vi "Distribution Example 2014yr.vi"() -> ()   [LabVIEW 2014]
uses:
  <vilib>/addons/database/Connection.llb/DB Tools Open Connec (Path).vi
  <userlib>/_OpenG.lib/array/array.llb/Search 1D Array (I32)__ogtk.vi
  <userlib>/_OpenG.lib/array/array.llb/Search 1D Array (Boolean)__ogtk.vi
  <vilib>/addons/database/NI_Database_API.lvlib
panel:
  out "size(s)":i32
  out "sum":i32
  out "Annual Distribution":cluster{dbl[], dbl[]}[](graph)
  out "Table 2":string[][](table)=[["34", "74", "23", "35", "23", "26", "74", "74", "21", "39", "61", "83"], ["73", "24", "75", "87", "42", "34", "35", "76", "52", "43", "43", "3"], ["36", "25", "12", "34", "24", "74", "73", "54", "88", "64", "90", "62"]]
  out "output array":i32[](array[numeric])
  out "Array 2":i32[](array[numeric])
  out "Array":i32[](array[numeric])
  out "data":string[][](table)
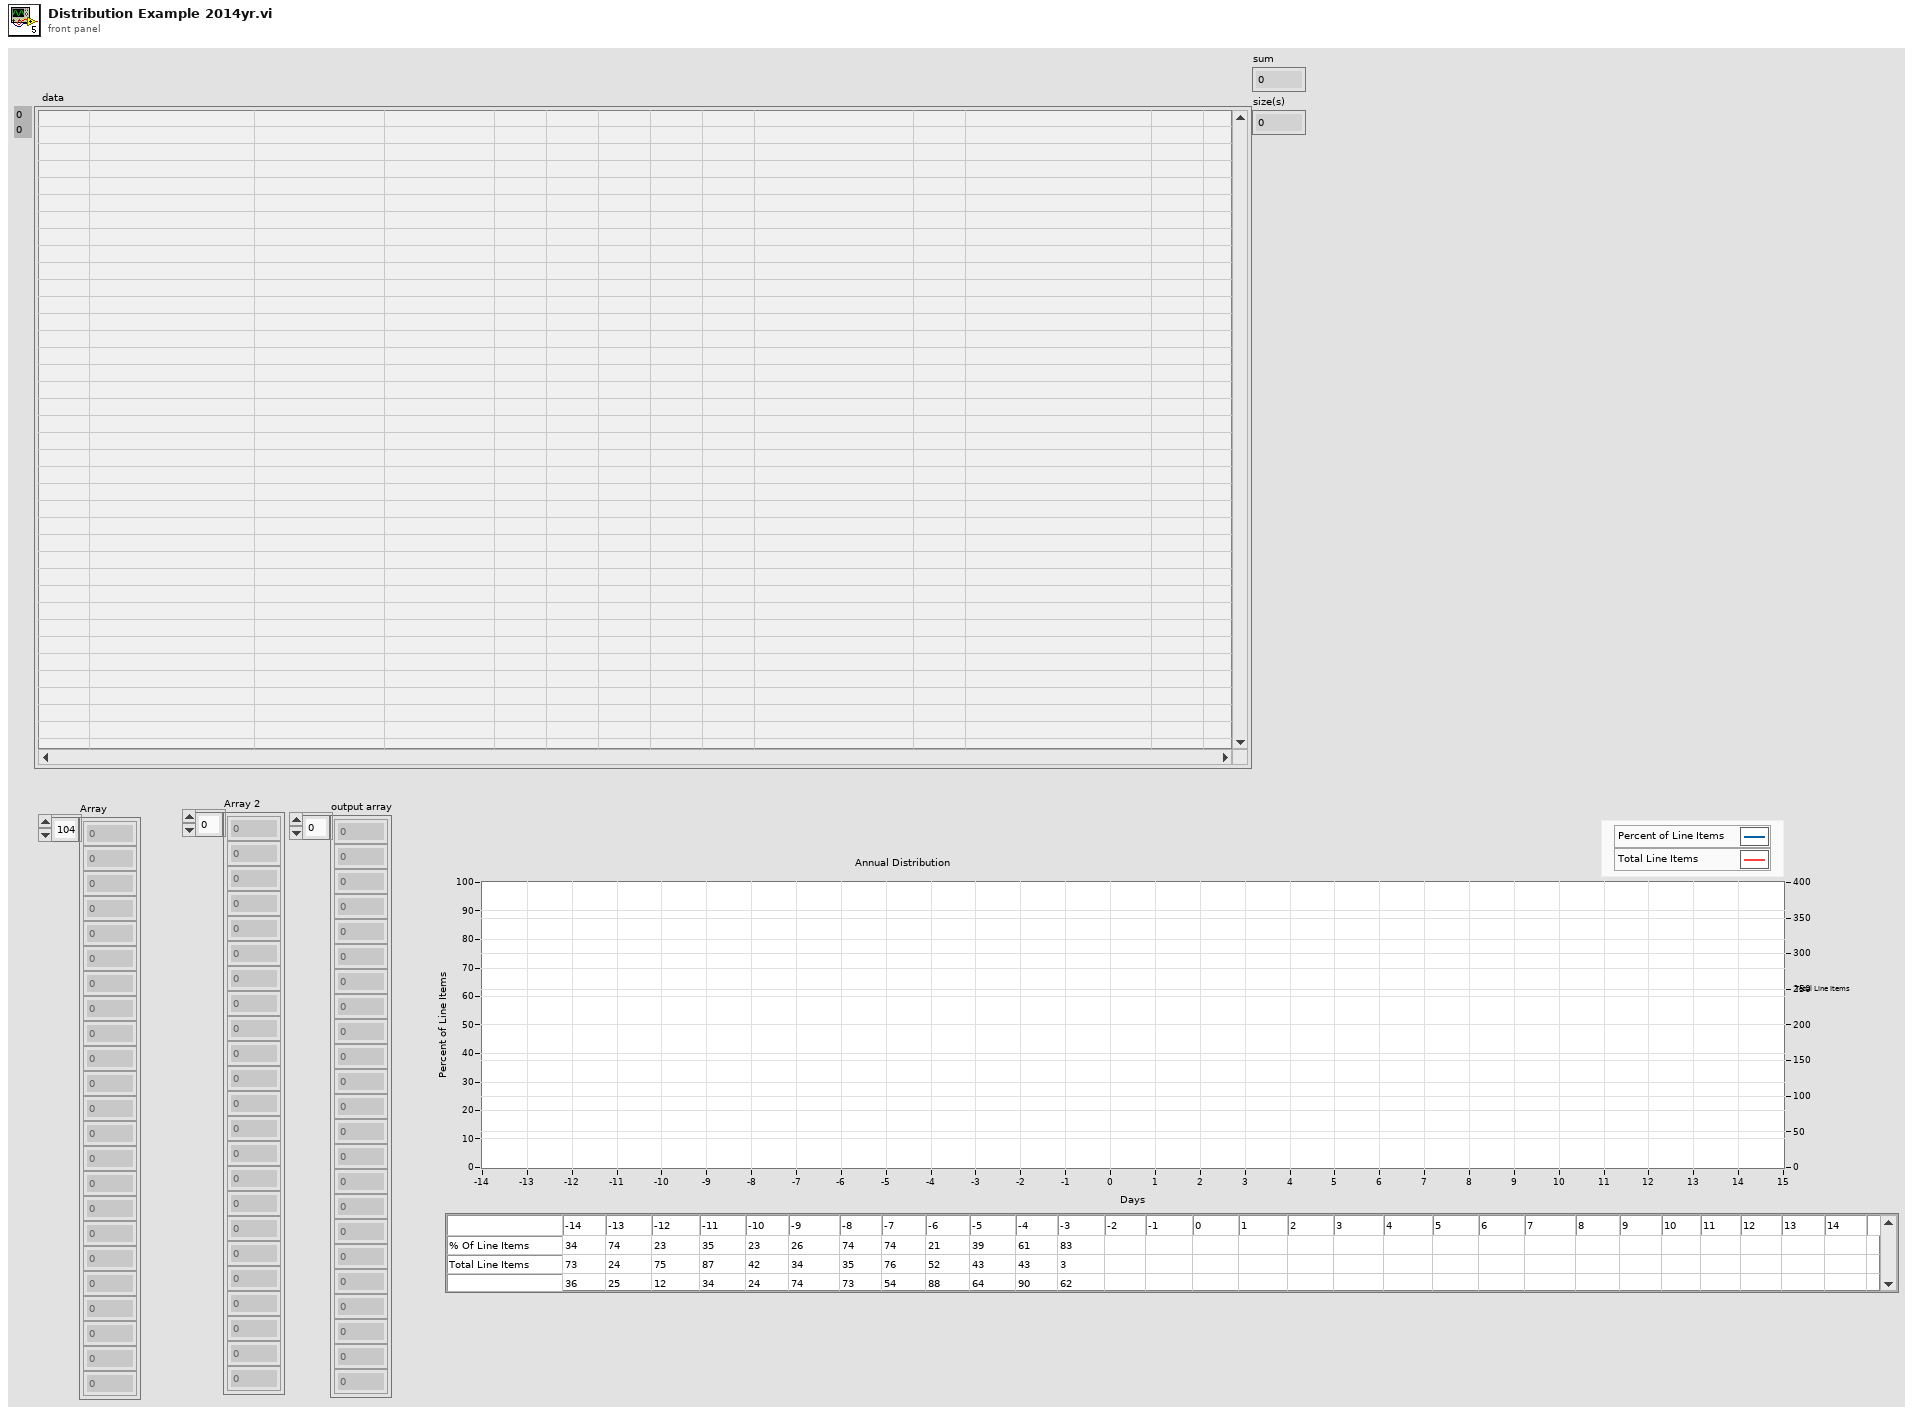
[diagram p1: front panel]
types:
  T1 = typedef "NI_Database_API.lvlib/Conn ObjectReference.ctl" = refnum<k1>
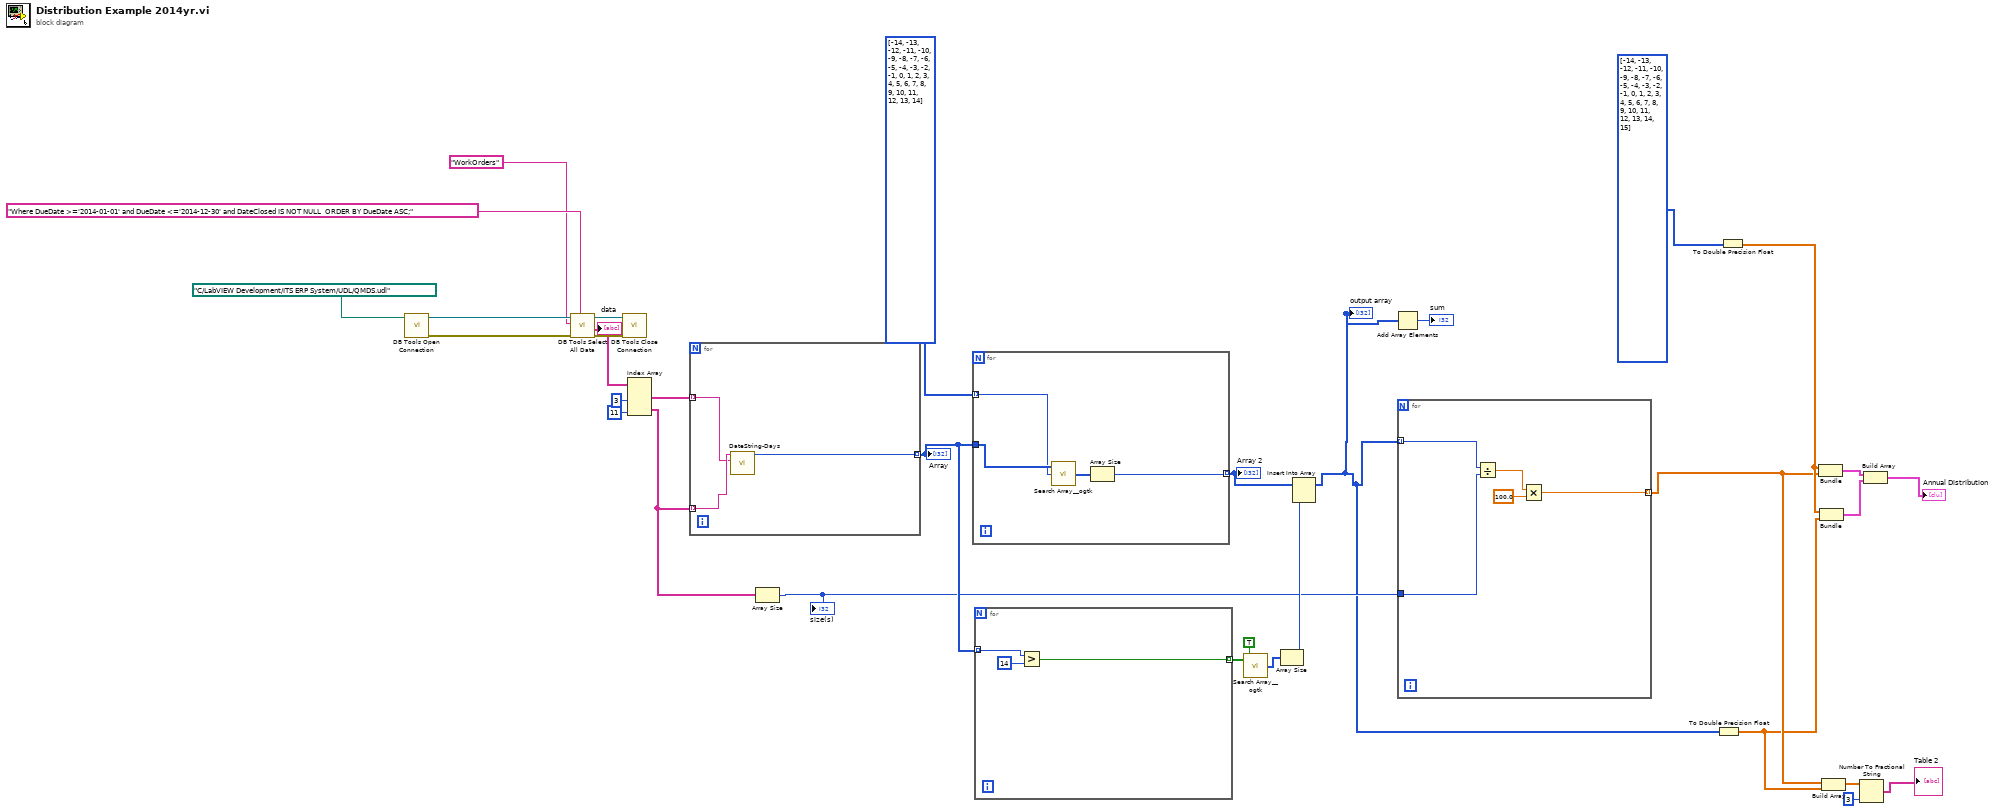
[diagram p0: block diagram]
diagram:
  n1 = call-poly <vilib>:"DB Tools Open Connection.vi"("connection information"=path "C:/LabVIEW Development/ITS ERP System/UDL/QMDS.udl" ("Database (mdb)  File Path")) -> ("error out"=w30:errorcluster, "connection reference"=w31:T1)  [unwired: 7 in]
  n2 = call <vilib>:"DB Tools Select All Data.vi"("optional clause"="Where DueDate >='2014-01-01' and DueDate <='2014-12-30' and DateClosed IS NOT NULL  ORDER BY DueDate ASC;", "error in (no error)"=w30, "table"="WorkOrders" ("Table"), "connection reference"=w31) -> ("error out"=w26:errorcluster, "data"=w25:string[][], "connection reference out"=w27:T1)  [unwired: 2 in]
  "data" <- w25
  n3 = call <vilib>:"DB Tools Close Connection.vi"("error in (no error)"=w26, "connection reference"=w27) -> ()  [unwired: 5 in, 1 out]
  n4 = Index Array(array=w25, index (col) #1=3 ("disabled index (col)"), index (col) #2=11 ("index (col)")) -> (element #1=w22:string[], element #2=w14:string[])  [unwired: 2 in]
  n5 = for {
    tunnel: w22 -> [w33] mode=indexing
    tunnel: w14 -> [w34] mode=indexing
    tunnel: [w35] -> w20 mode=indexing
    n6 = call "DateString-Days.vi"("First date"=w33, "Second date"=w34) -> ("Elapsed days"=w35:i32)  [unwired: 8 in, 1 out]
  }
  "Array" <- w20
  n7 = Array Size(array=w14) -> (size(s)=w13:i32)
  "size(s)" <- w13
  n8 = for {
    tunnel: i32[] [-14, -13, -12, -11, -10, -9, -8, -7, -6, -5, -4, -3, -2, -1, 0, 1, 2, 3, 4, 5, 6, 7, 8, 9, 10, 11, 12, 13, 14] -> [w38] mode=indexing
    tunnel: w20 -> [w39]
    tunnel: [w36] -> w19 mode=indexing
    n9 = call-poly <userlib>:"Search Array__ogtk.vi"("Array"=w39, "Element Data"=w38) -> ("Indices of Elements"=w37:i32[])  [unwired: 7 in]
    n10 = Array Size(array=w37) -> (size(s)=w36:i32)
  }
  "Array 2" <- w19
  n11 = for {
    tunnel: w20 -> [w40] mode=indexing
    tunnel: [w41] -> w17 mode=indexing
    n12 = Greater?(x=w40, y=14) -> (0:w41:bool)
  }
  n13 = call-poly <userlib>:"Search Array__ogtk.vi"("Array"=w17, "Element Data"=TRUE) -> ("Indices of Elements"=w15:i32[])  [unwired: 7 in]
  n14 = Array Size(array=w15) -> (size(s)=w18:i32)
  n15 = Insert Into Array(array=w19, new element=w18) -> (w1:i32[])  [unwired: 1 in]
  "output array" <- w1
  n16 = Add Array Elements(numeric array=w1) -> (sum=→"sum":i32)
  n17 = for {
    tunnel: w1 -> [w47] mode=indexing
    tunnel: w13 -> [w46]
    tunnel: [w43] -> w8 mode=indexing
    n18 = Divide(x=w47, y=w46) -> (x/y=w45:dbl)
    n19 = Multiply(x=w45, y=100.0) -> (x*y=w43:dbl)
  }
  n20 = To Double Precision Float(number=w1) -> (double precision float=w7:dbl[])
  n21 = To Double Precision Float(number=i32[] [-14, -13, -12, -11, -10, -9, -8, -7, -6, -5, -4, -3, -2, -1, 0, 1, 2, 3, 4, 5, 6, 7, 8, 9, 10, 11, 12, 13, 14, 15]) -> (double precision float=w12:dbl[])
  n22 = Bundle(w12, w8) -> (w11:cluster{dbl[], dbl[]})  [unwired: 1 in]
  n23 = Bundle(w12, w7) -> (w10:cluster{dbl[], dbl[]})  [unwired: 1 in]
  n24 = Build Array(w8, w7) -> (w6:dbl[][])
  n25 = Number To Fractional String(number=w6, precision (6)=i16 3) -> (F-format string=→"Table 2":string[][])  [unwired: 2 in]
  n26 = Build Array(w11, w10) -> (→"Annual Distribution":cluster{dbl[], dbl[]}[])
